vi "Builder.AddToProject.vi"(7 "App.Instance (this app)":refnum<vi>, 8 "error in":errorcluster, 10 "File Path":path, 11 "Project Path":path) -> (0 "error out":errorcluster)   [LabVIEW 2011]
doc: "This VI adds the reference <B>file</B> to the given <B>project</B>.\nThe project must be opnenend in the <B>App.Instance</B>"
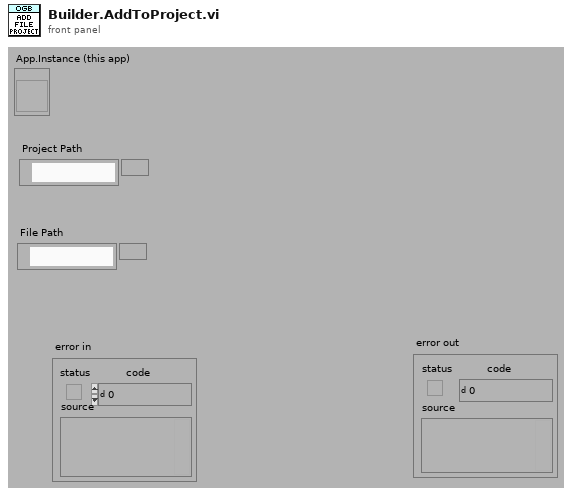
[diagram p1: front panel]
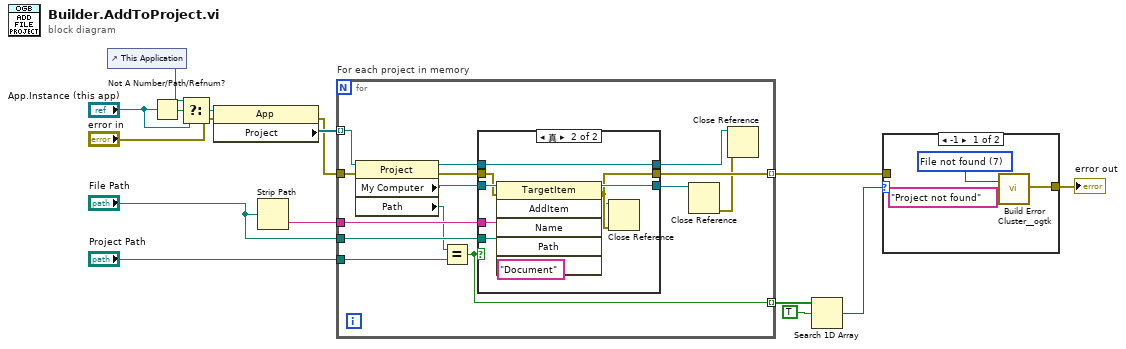
[diagram p0: block diagram]
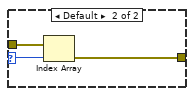
[diagram p2: hidden frame]
diagram:
  n1 = control-ref of="This Application"() -> (w1:refnum<vi>)
  n2 = Not A Number/Path/Refnum?(number/path/refnum="App.Instance (this app)") -> (NaN/Path/Refnum?=w4:bool)
  n3 = Select(t=w1, s=w4, f="App.Instance (this app)") -> (s? t:f=w2:refnum<vi>)
  n4 = property class="App"(reference=w2, error in="error in") -> (error out=w12:errorcluster, "Project"=w15:refnum<vi>[])  [unwired: 1 out]
  n5 = Strip Path(path="File Path") -> (name=w13:string)  [unwired: 1 out]
  n6 = for "For each project in memory" {
    tunnel: "File Path" -> [w25]
    tunnel: [w20] -> w7 mode=indexing
    tunnel: w15 -> [w27] mode=indexing
    tunnel: w13 -> [w26]
    tunnel: w12 -> [w24]
    tunnel: "Project Path" -> [w22]
    tunnel: [w16] -> w9 mode=indexing
    n7 = property class="Project"(reference=w27, error in=w24) -> (reference out=w21:refnum<vi>, error out=w28:errorcluster, "My Computer"=w29:refnum<vi>, "Path"=w23:path)
    n8 = Equal?(x=w23, y=w22) -> (x = y?=w16:bool)
    n9 = case shown="真" w16 {
      tunnel: w29 -> [w30 w41]
      tunnel: w28 -> [w31 w40]
      tunnel: [w31 w35] -> w20
      tunnel: w26 -> [_ w39]
      tunnel: w25 -> [_ w38]
      tunnel: [w32 w37] -> w17
      tunnel: w21 -> [w32 w37]
      tunnel: [w30 w36] -> w19
      frame False {
      }
      frame True {
        n10 = invoke class="TargetItem" method="AddItem"(reference=w41, error in=w40, "Name"=w39, "Path"=w38, "Type"="Document") -> (reference out=w36:refnum<vi>, error out=w35:errorcluster, "AddItem"=w34:refnum<vi>)  [unwired: 1 in, 3 out]
        n11 = Close Reference(reference=w34, error in (no error)=w35) -> ()  [unwired: 1 out]
      }
    }
    n12 = Close Reference(reference=w19) -> (error out=w18:errorcluster)  [unwired: 1 in]
    n13 = Close Reference(reference=w17, error in (no error)=w18) -> ()  [unwired: 1 out]
  }
  n14 = Search 1D Array(1D array=w9, element=TRUE) -> (index of element=w5:i32)  [unwired: 1 in]
  n15 = case shown="-1" w5 {
    selector: w5 -> [_ w45]
    tunnel: w7 -> [_ w47]
    tunnel: [w44 w46] -> w6
    frame -1 {
      w43 = 7 items=["No error", "Argument error", "Memory is full", "Out of zone", "End of file", "File already open", "Generic file I/O error", "File not found", "File permission error", "Disk is full", "Duplicate path", "Too many files open", "System feature not enabled", "Resource file not found", "Cannot add resource", "Resource not found", "Image not found", "Image memory error", "Pen does not exist", "Config type invalid", "Config token not found", "Config parse error", "Config memory error", "Bad external code format", "Bad external code offset", "External code not present", "Null window", "Destroy window error", "Null menu", "Print aborted", "Bad print record", "Print driver error", "Windows error during printing", "Memory error during printing", "Print dialog error", "Generic print error", "Invalid device refnum", "Device not found", "Device parameter error", "Device unit error", "Cannot open device", "Device call aborted", "Generic error", "Cancelled by user", "Object ID too low", "Object ID too high", "Object not in heap", "Unknown heap", "Unknown object (invalid DefProc)", "Unknown object (DefProc not in table)", "Message out of range", "Invalid (null) method", "Unknown message", "Manager call not supported", "Bad address", "Network operation in progress", "Network operation timed out", "Connection is busy", "Network attribute not supported", "Network error", "Address in use", "System out of memory", "Connection aborted", "Connection refused", "Not connected", "Already connected", "Connection closed", "Initialization error (interapplication manager)", "Bad occurrence", "Wait on unbound occurrence handler", "Occurrence queue overflow", "Datalog type conflict", "Unused", "Unrecognized type (interapplication manager)", "Memory corrupt", "Failed to make temporary DLL", "Old CIN version", "Drag socket not found", "Failed to load drop-object", "Failed to register OLE object", "Failed to release OLE object", "Format specifier type mismatch", "Unknown format specifier", "Too few format specifiers", "Too many format specifiers", "Scan failed", "Newer CIN version", "Error converting to variant", "Runtime menu error", "Password tampered", "Variant attribute not found", "Incompatible variant data type", "Event data is not available", "Event Store is not present", "Occurrence is not found", "Event Queue is not created", "Event info is not available", "Refnum passed is NULL", "Error retrieving Class GUID", "Error retrieving CoClass GUID", "Error retrieving TypeLib GUID.", "Bad built application magic bytes.", "Specific driver is different from the specific driver associated with the Logical Name.", "There is no session opened to the class driver.", "Max Error", "MAX - Error with config objects", "MAX - Error loading configuration", "MAX - Group not supported"]
      n16 = call <userlib>:"Build Error Cluster__ogtk.vi"("String to Prepend to source (\"\")"="Project not found" ("String to Prepend to source (\"\")"), "code"=w43) -> ("error out"=w44:errorcluster)
    }
    frame Default {
      n17 = Index Array(array=w47, index=w45) -> (element=w46:errorcluster)
    }
  }
  "error out" <- w6
